vi "Build.vi"(4 "Timeout_ms":i32, 5 "HttpResponseMessage in":refnum<class "HttpResponseMessage.lvclass">, 6 "NET_CancellationSource":refnum<k24>, 8 "error in (no error)":errorcluster, 11 "NET_HttpResponseMessage":refnum<k24>) -> (0 "error out":errorcluster, 3 "HttpResponseMessage out":refnum<class "HttpResponseMessage.lvclass">)   [LabVIEW 2018, in "HttpClient_NET.lvlib" / "HttpResponseMessage.lvclass"]
doc: "<b> </b> <b> </b>\nHttpClient_NET\nJustin Young - Viviota\nCopyright (c) 2021\nLicense: BSD"
uses:
  HttpResponseMessage.lvclass
  HttpResponseMessage.lvclass/HttpResponseMessage.ctl
  Accessors/Write NET_HttpResponseTask.vi
  Accessors/Write NET_CancellationSource.vi
  Accessors/Write Timeout_ms.vi
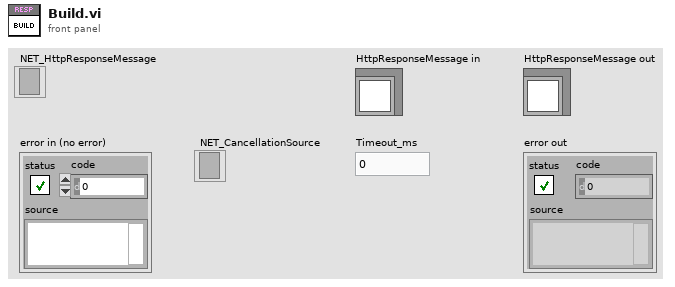
[diagram p1: front panel]
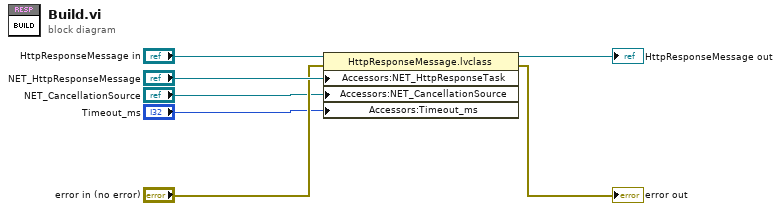
[diagram p0: block diagram]
diagram:
  n1 = property class="HttpResponseMessage.lvclass"(reference="HttpResponseMessage in", error in="error in (no error)", "Accessors:NET_HttpResponseTask"="NET_HttpResponseMessage", "Accessors:NET_CancellationSource"="NET_CancellationSource", "Accessors:Timeout_ms"="Timeout_ms") -> (reference out=→"HttpResponseMessage out":refnum<class "HttpResponseMessage.lvclass">, error out=→"error out":errorcluster)
